vi "add parameter indicies controls.vi"(8 "error in":errorcluster, 9 "Channels to create":T1[](array[typedef]), 10 "cfg class path":path, 11 "Application in":refnum<vi>) -> (0 "error out":errorcluster)   [LabVIEW 2013, in "FixedChannelTBModuleDecideFeatures.lvclass"]
uses:
  FixedChannelTBModuleDecideFeatures.lvclass
  channel configuration.ctl
  <vilib>/NI/Tag Bus Module Framework/channel/channel classification.ctl
  <vilib>/NI/Tag Bus/tag/Data Type.ctl
  <vilib>/NI/Tag Bus Module Framework/channel/TBM channel.lvclass
  <vilib>/NI/Tag Bus/tag/tag descriptor.lvclass
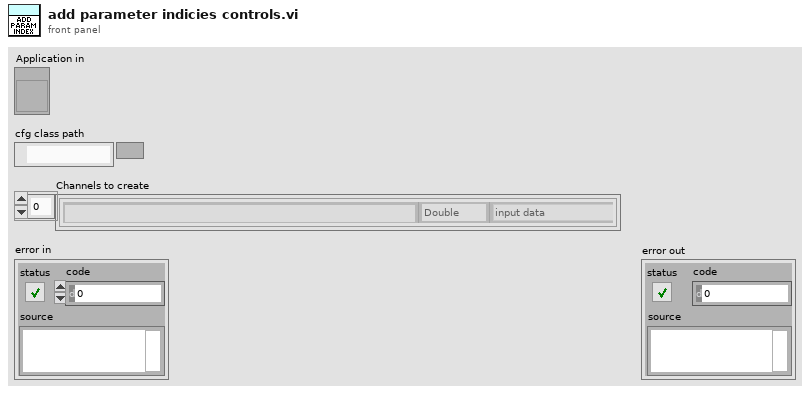
[diagram p1: front panel]
types:
  T1 = typedef "FixedChannelTBModuleDecideFeatures.lvclass/channel configuration.ctl" = cluster{"Name":string, "channel classification":T2, "data type":T3}
  T2 = typedef "TBM channel.lvclass/channel classification.ctl" = enum16{"input data", "output data", "processing parameter", "processing result"}
  T3 = typedef "tag bus.lvlib/tag descriptor.lvclass/Data Type.ctl" = enum16{"Double", "Single", "I64", "I32", "I16", "I8", "U64", "U32", "U16", "U8", "Boolean", "String", "Array of Double", "Array of Single", "Array of I64", "Array of I32", "Array of I16", "Array of I8", "Array of U64", "Array of U32", "Array of U16", "Array of U8", "Array of Boolean", "Array of String"}
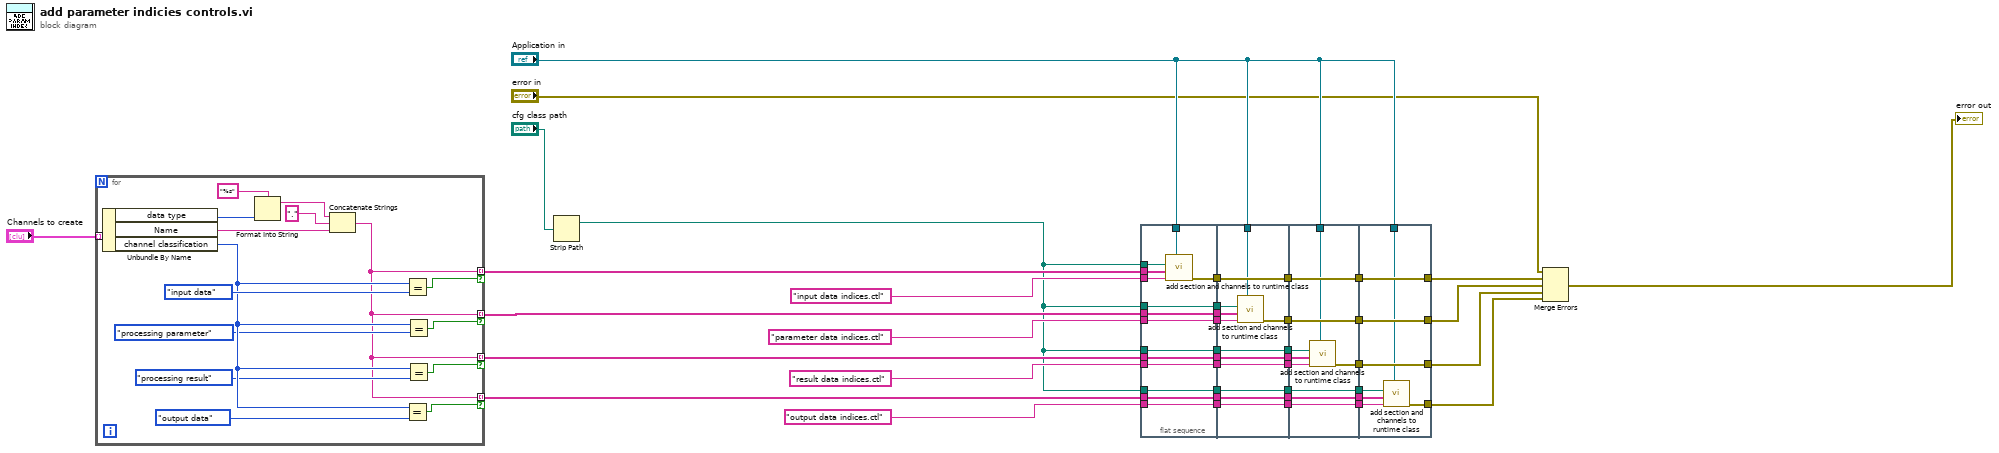
[diagram p0: block diagram]
diagram:
  n1 = for {
    tunnel: "Channels to create" -> [w58] mode=indexing
    tunnel: [w44] -> w39 mode=indexing if=w56
    tunnel: [w44] -> w36 mode=indexing if=w55
    tunnel: [w44] -> w28 mode=indexing if=w53
    tunnel: [w44] -> w20 mode=indexing if=w54
    n2 = Unbundle By Name(w58) -> ("data type"=w48:T3, "Name"=w46:string, "channel classification"=w52:T2)
    n3 = Format Into String(format string="%s", w48) -> (resulting string=w47:string)  [unwired: 2 in, 1 out]
    n4 = Concatenate Strings(w47, "." ("string"), w46) -> (w44:string)
    n5 = Equal?(x=w52, y=channel_classification."output data" ("x")) -> (x = y?=w54:bool)
    n6 = Equal?(x=w52, y=channel_classification."input data" ("x")) -> (x = y?=w56:bool)
    n7 = Equal?(x=w52, y=channel_classification."processing parameter" ("x")) -> (x = y?=w55:bool)
    n8 = Equal?(x=w52, y=channel_classification."processing result" ("x")) -> (x = y?=w53:bool)
  }
  n9 = Strip Path(path="cfg class path") -> (stripped path=w21:path)  [unwired: 1 out]
  n10 = flat-sequence {
    tunnel: w39 -> [w72]
    tunnel: "input data indices.ctl" ("name or relative path") -> [w71]
    tunnel: w21 -> [w70]
    tunnel: [w69] -> w37
    tunnel: w21 -> [w69]
    tunnel: w36 -> [w68]
    tunnel: [w68] -> w35
    tunnel: [w67] -> w34
    tunnel: "parameter data indices.ctl" ("name or relative path") -> [w67]
    tunnel: [w66] -> w31
    tunnel: w21 -> [w66]
    tunnel: [w65] -> w29
    tunnel: w28 -> [w65]
    tunnel: "result data indices.ctl" ("name or relative path") -> [w64]
    tunnel: [w64] -> w25
    tunnel: [w63] -> w22
    tunnel: w21 -> [w63]
    tunnel: w20 -> [w62]
    tunnel: [w62] -> w19
    tunnel: [w61] -> w14
    tunnel: "output data indices.ctl" ("name or relative path") -> [w61]
    tunnel: [w60] -> w9
    tunnel: "Application in" -> [w59]
    tunnel: w37 -> [w84]
    tunnel: w35 -> [w83]
    tunnel: w34 -> [w82]
    tunnel: [w81] -> w32
    tunnel: w31 -> [w81]
    tunnel: [w80] -> w30
    tunnel: w29 -> [w80]
    tunnel: [w79] -> w26
    tunnel: w25 -> [w79]
    tunnel: [w78] -> w23
    tunnel: w22 -> [w78]
    tunnel: w19 -> [w77]
    tunnel: [w77] -> w18
    tunnel: [w76] -> w15
    tunnel: w14 -> [w76]
    tunnel: [w75] -> w10
    tunnel: w9 -> [w75]
    tunnel: [w74] -> w7
    tunnel: "Application in" -> [w73]
    tunnel: w32 -> [w94]
    tunnel: w30 -> [w93]
    tunnel: w26 -> [w92]
    tunnel: [w91] -> w24
    tunnel: w23 -> [w91]
    tunnel: w18 -> [w90]
    tunnel: [w90] -> w17
    tunnel: [w89] -> w16
    tunnel: w15 -> [w89]
    tunnel: [w88] -> w11
    tunnel: w10 -> [w88]
    tunnel: [w87] -> w8
    tunnel: w7 -> [w87]
    tunnel: [w86] -> w6
    tunnel: "Application in" -> [w85]
    tunnel: w24 -> [w102]
    tunnel: w17 -> [w101]
    tunnel: w16 -> [w100]
    tunnel: [w99] -> w12
    tunnel: w11 -> [w99]
    tunnel: [w98] -> w5
    tunnel: w8 -> [w98]
    tunnel: [w97] -> w4
    tunnel: w6 -> [w97]
    tunnel: [w96] -> w3
    tunnel: "Application in" -> [w95]
    frame #0 {
      n11 = call "add section and channels to runtime class.vi"("Application in"=w59, "Typedef relative path"=w71, "channels"=w72, "cfg class base path"=w70) -> ("error out"=w60:errorcluster)  [unwired: 7 in]
    }
    frame #1 {
      n12 = call "add section and channels to runtime class.vi"("Application in"=w73, "Typedef relative path"=w82, "channels"=w83, "cfg class base path"=w84) -> ("error out"=w74:errorcluster)  [unwired: 7 in]
    }
    frame #2 {
      n13 = call "add section and channels to runtime class.vi"("Application in"=w85, "Typedef relative path"=w92, "channels"=w93, "cfg class base path"=w94) -> ("error out"=w86:errorcluster)  [unwired: 7 in]
    }
    frame #3 {
      n14 = call "add section and channels to runtime class.vi"("Application in"=w95, "Typedef relative path"=w100, "channels"=w101, "cfg class base path"=w102) -> ("error out"=w96:errorcluster)  [unwired: 7 in]
    }
  }
  n15 = Merge Errors("error in", w12, w5, w4, w3) -> (→"error out":errorcluster)
